vi "DriveExecute_PID_Autotune.vi"(8 "error in (no error)":errorcluster) -> (0 "error out":errorcluster)   [LabVIEW 2020]
doc: "Execute for Drie\n\nClosed control loop for drive\n\ninput: \n error in (cluster)\n\noutput:\n error out (cluster)"
uses:
  <vilib>/Rock Robotics/WPI/ThirdParty/Phoenix-LabVIEW/Motor Controller/Controls/CTRE_Phoenix_MotorControl_ControlMode.ctl
  <vilib>/Rock Robotics/WPI/ThirdParty/JAS_Junk/TrajLib/SimpleMotorFF_Calculate.vi
  <vilib>/Rock Robotics/WPI/ThirdParty/JAS_Junk/TrajLib/VI/Util_GetTime_U32.vi
  <vilib>/Rock Robotics/WPI/ThirdParty/JAS_Junk/TrajLib/PIDController_AtSetpoint.vi
  <vilib>/Rock Robotics/WPI/ThirdParty/JAS_Junk/TrajLib/PIDController_SetPIDF.vi
  <vilib>/Rock Robotics/WPI/ThirdParty/JAS_Junk/TrajLib/PIDController_SetDerivativeFilter.vi
  <vilib>/Rock Robotics/WPI/ThirdParty/JAS_Junk/TrajLib/PIDController_SetIntegratorRange.vi
  <vilib>/Rock Robotics/WPI/ThirdParty/JAS_Junk/TrajLib/PIDController_SetTolerancePandV.vi
  <vilib>/Rock Robotics/WPI/ThirdParty/JAS_Junk/TrajLib/PIDController_DisableContinousInput.vi
  <vilib>/Rock Robotics/WPI/ThirdParty/JAS_Junk/TrajLib/PIDController_EnableContinousInput.vi
  <vilib>/Rock Robotics/WPI/ThirdParty/JAS_Junk/TrajLib/PIDController_Reset.vi
  <vilib>/Rock Robotics/WPI/ThirdParty/JAS_Junk/TrajLib/PIDController_New.vi
  <vilib>/Rock Robotics/WPI/ThirdParty/JAS_Junk/TrajLib/PIDController_SetOutputLimits.vi
  <vilib>/Rock Robotics/WPI/ThirdParty/JAS_Junk/TrajLib/SlewRateLimiter_New.vi
  <vilib>/Rock Robotics/WPI/ThirdParty/JAS_Junk/TrajLib/SlewRateLimiter_Reset.vi
  <vilib>/Rock Robotics/WPI/ThirdParty/JAS_Junk/TrajLib/SlewRateLimiter_Calculate.vi
  <vilib>/Rock Robotics/WPI/ThirdParty/JAS_Junk/TrajLib/SlewRateLimiter_SetRate.vi
  <vilib>/Rock Robotics/WPI/ThirdParty/JAS_Junk/TrajLib/PIDController_NewPeriod.vi
  <vilib>/Rock Robotics/SystemInterfaces/NetworkCommunication/NetComm_UsageReport_report.vi
  <vilib>/Rock Robotics/SystemInterfaces/Utilities/FPGA_UtilitiesRead LocalTime.vi
  <vilib>/Rock Robotics/WPI/ThirdParty/JAS_Junk/TrajLib/VI/Util_GetTime_U64.vi
  DriveGlobal.vi
  <vilib>/Rock Robotics/WPI/ThirdParty/Phoenix-LabVIEW/Motor Controller/Get/CTRE_Phoenix_MotorController_GetSelectedSensorData.vi
  <vilib>/Rock Robotics/WPI/ThirdParty/JAS_Junk/TrajLib/Globals/Util_LibraryGlobals.vi
  <vilib>/Rock Robotics/WPI/ThirdParty/JAS_Junk/TrajLib/PIDController_AdvCalculate_FF_Sp_Pv.vi
  <vilib>/Rock Robotics/Network Tables/NT Write Value.vi
  <vilib>/Rock Robotics/Network Tables/NT Write Boolean.vi
  <vilib>/Rock Robotics/Network Tables/NT Write Number.vi
  <vilib>/Rock Robotics/WPI/ThirdParty/JAS_Junk/TrajLib/Trajectory_Library.lvlib
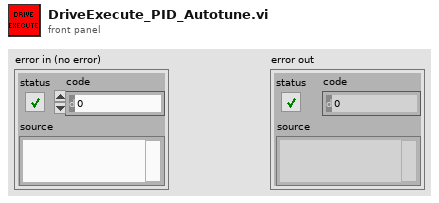
[diagram p1: front panel]
types:
  T1 = enum16{"Ziegler Nicols - Fast", "Ziegler Nicols - Normal", "Ziegler Nicols - Slow", "CHR regulator - 0% overshoot", "CHR regulator - 20% overshoot", "CHR servo - 0 % overshoot", "CHR servo - 20% overshoot"}
  T2 = typedef "CTRE_Phoenix_MotorControl_ControlMode.ctl" = u16
  T3 = typedef "WPI_MotorControlDeviceRef.ctl" = cluster{"DeviceStatus":errorcluster, "Type":T4, "PWM":cluster{"PWM Channel":T5, "DeadBand":T6}, "CAN":cluster{"Device Number":u8, "SetOutput VI Ref":variant, "GetOutput VI Ref":variant, "Enable VI Ref":variant, "Disable VI Ref":variant, "Data":variant}, "Invert":bool, "DIO PWM":cluster{"PWM \"Enable\" Channel":T5, "DIOChannel":T7, "PWM Rate":dbl}}
  T4 = typedef "WPI_MotorControlType.ctl" = enum16{"PWM", "CAN", "DIO PWM"}
  T5 = typedef "FPGA_DIOPWMChannel.ctl" = enum8{"PWM 0", "PWM 1", "PWM 2", "PWM 3", "PWM 4", "PWM 5", "PWM 6", "PWM 7", "PWM 8", "PWM 9", "PWM MXP 0", "PWM MXP 1", "PWM MXP 2", "PWM MXP 3", "PWM MXP 4", "PWM MXP 5", "PWM MXP 6", "PWM MXP 7", "PWM MXP 8", "PWM MXP 9", "Invalid"}
  T6 = typedef "WPI_PWMDeadband.ctl" = cluster{"Name":string, "maxPositivePwm":i32, "minPositivePwm":i32, "centerPwm":i32, "maxNegativePwm":i32, "minNegativePwm":i32, "angularRange":u16}
  T7 = typedef "FPGA_DIOChannel.ctl" = enum8{"DIO 0", "DIO 1", "DIO 2", "DIO 3", "DIO 4", "DIO 5", "DIO 6", "DIO 7", "DIO 8", "DIO 9", "DIO MXP 0", "DIO MXP 1", "DIO MXP 2", "DIO MXP 3", "DIO MXP 4", "DIO MXP 5", "DIO MXP 6", "DIO MXP 7", "DIO MXP 8", "DIO MXP 9", "DIO MXP 10", "DIO MXP 11", "DIO MXP 12", "DIO MXP 13", "DIO MXP 14", "DIO MXP 15", "SPI Port CS1", "SPI Port CS2", "SPI Port CS3", "SPI Port MISO", "SPI Port MOSI", "Invalid"}
  T8 = typedef "ADIS16470 Device Reference.ctl" = cluster{"DevStatus":errorcluster, "Hardware Config":T9, "Calibration Complete":refnum<notifier>, "Status Reference":refnum<data-value>, "Data Reference":refnum<data-value>, "Sychronous Process VI":T12, "Cmd FIFO":refnum<k33>, "Source":T13, "Data FIFO":refnum<k33>, "Calibration Time (ms)":u32, "Data Reference":refnum<data-value>}
  T9 = typedef "ADIS16470 Hardware Configuration.ctl" = cluster{"SPI Clock Rate (Hz)":dbl, "IMU SPI Mode (3)":T10, "IMU Reset Pin":T7, "IMU SPI Bus":T11, "IMU Data Ready Pin":T7, "Stall Config":cluster{"Pow2BytesPerRead":u8, "StallTicks":u16, "CsToSclkTicks":u8}}
  T10 = typedef "WPI_SPIMode.ctl" = enum16{"Mode 0 (Clk Idle Low,Sample on Leading)", "Mode 1 (Clk Idle Low,Sample on Trailing)", "Mode 2 (Clk Idle High,Sample on Leading)", "Mode 3 (Clk Idle High,Sample on Trailing)"}
  T11 = typedef "spi_bus.ctl" = enum16{"SPI On-Board, CS0", "SPI On-Board, CS1", "SPI On-Board, CS2", "SPI On-Board, CS3", "SPI MXP", "Invalid"}
  T12 = typedef "ADIS16470 Process.ctl" = refnum<vi>
  T13 = typedef "FPGA_CounterEncoderSourceConvertionLVSourceType.ctl" = cluster{"DevStatus":errorcluster, "AnalogTriggerMode?":bool, "DigitalMode":cluster{"DIO Channel":T14}, "AnalogTriggerMode":cluster{"AnalogTriggerIndex":T15, "OutputType":T16}}
  T14 = typedef "FPGA_DIODigitalSourceChannel.ctl" = enum8{"DIO 0", "DIO 1", "DIO 2", "DIO 3", "DIO 4", "DIO 5", "DIO 6", "DIO 7", "DIO 8", "DIO 9", "DIO MXP 0", "DIO MXP 1", "DIO MXP 2", "DIO MXP 3", "DIO MXP 4", "DIO MXP 5", "DIO MXP 6", "DIO MXP 7", "DIO MXP 8", "DIO MXP 9", "DIO MXP 10", "DIO MXP 11", "DIO MXP 12", "DIO MXP 13", "DIO MXP 14", "DIO MXP 15", "SPI Port CS1", "SPI Port CS2", "SPI Port CS3", "SPI Port MISO", "SPI Port MOSI", "Disabled"}
  T15 = typedef "FPGA_AnalogTriggerIndex.ctl" = enum8{"Trig 0", "Trig 1", "Trig 2", "Trig 3", "Trig 4", "Trig 5", "Trig 6", "Trig 7", "Invalid"}
  T16 = typedef "FPGA_AnalogTriggerOutType.ctl" = enum16{"InWindow", "TriggerState", "Rising", "Falling"}
  T17 = typedef "ADIS16470 Data.ctl" = cluster{"XAngle":dbl, "YAngle":dbl, "ZAngle":dbl}
  T18 = typedef "Trajectory_Library.lvlib/SIMPLE_MOTOR_FF.ctl" = cluster{"Ks":dbl, "Kv":dbl, "Ka":dbl, "KnInv":dbl}
  T19 = typedef "Trajectory_Library.lvlib/PID_ADV_LIMITS.ctl" = cluster{"MaxInput":dbl, "MinInput":dbl, "Continuous":bool, "MaxOutput":dbl, "MinOutput":dbl}
  T20 = typedef "Trajectory_Library.lvlib/PID_ADV_TUNING.ctl" = cluster{"Kf":dbl, "Kp":dbl, "Ki":dbl, "Kd":dbl, "MaximumIntegral":dbl, "MinimumIntegral":dbl, "Filter Derivative":bool}
  T21 = cluster{"Controller Constant Type":enum16{"Ziegler Nicols - Fast", "Ziegler Nicols - Normal", "Ziegler Nicols - Slow", "CHR regulator - 0% overshoot", "CHR regulator - 20% overshoot", "CHR servo - 0 % overshoot", "CHR servo - 20% overshoot"}, "Type of Controller":enum16{"P", "PI", "PID"}, "CO Offset":dbl, "Kn":dbl, "Tuning Tolerance":dbl, "Plant Tolerance":dbl, "Newest Avg Time ":i32, "Long Ave Time":i32}
  T22 = cluster{"Plant Gain (K)":dbl, "Time Constant (T)":dbl, "Dead Time (L)":dbl, "stimulus operating point":dbl, "response operating point":dbl}
  T23 = cluster{"proportional gain (Kp)":dbl, "integral time (Ki / Sec)":dbl, "derivative time (Kd /Sec)":dbl}
  T24 = cluster{"Const Done":bool, "Plant Done":bool, "PV Std Dev":dbl, "CO Std Dev":dbl}
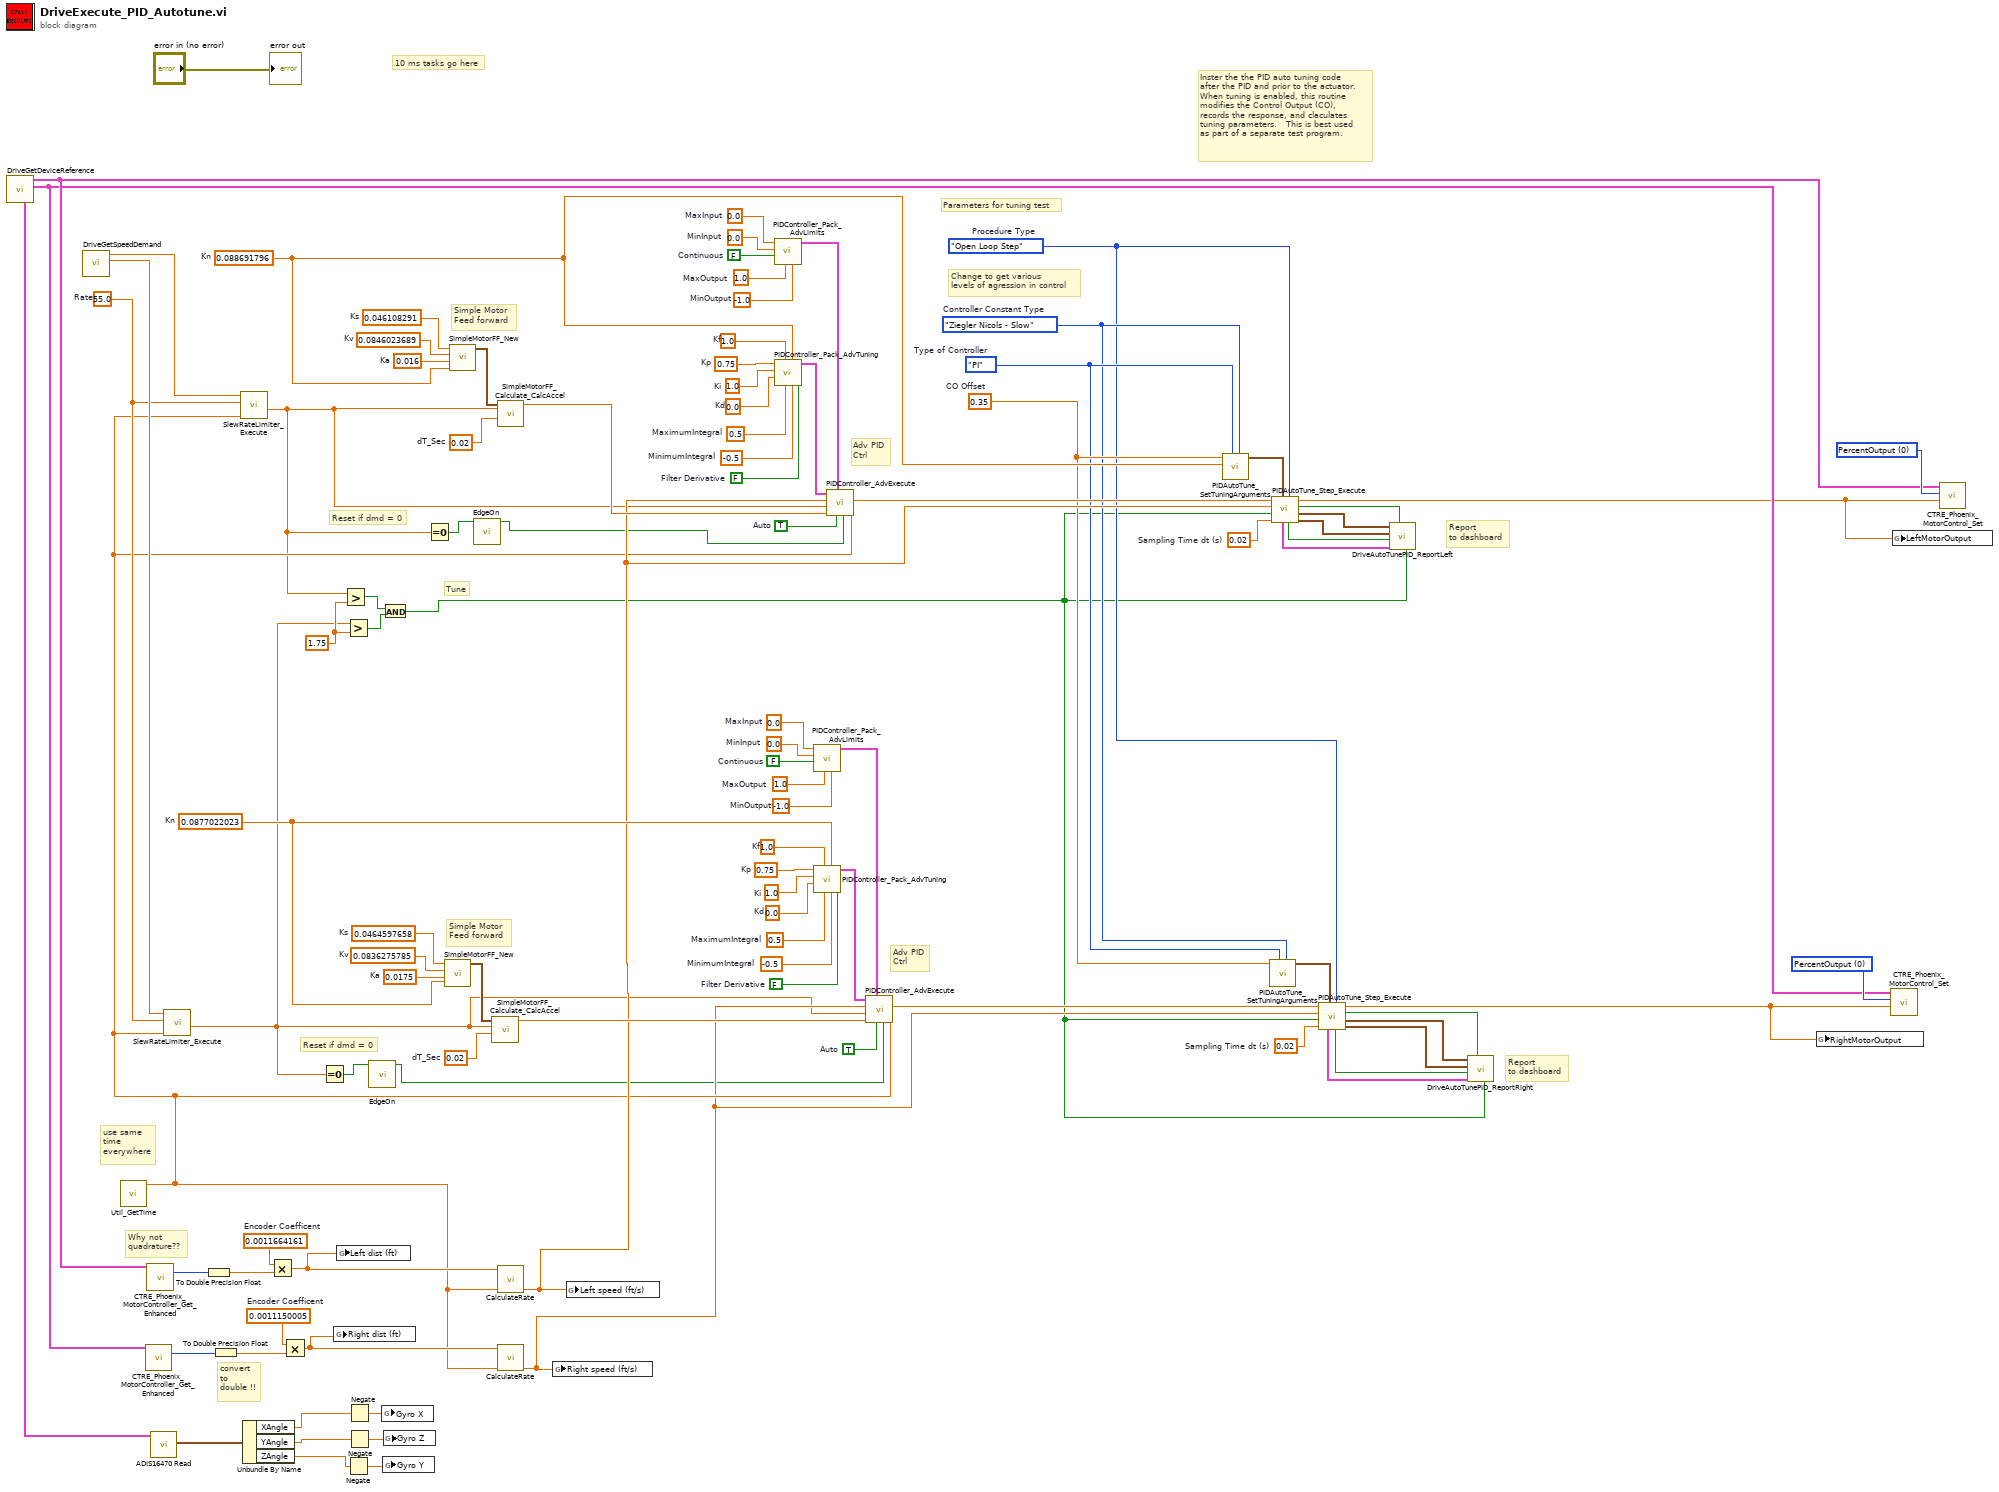
[diagram p0: block diagram]
diagram:
  w24 = enum16{"Open Loop Step", "Closed Loop Step"}."Open Loop Step"  # Procedure Type
  w25 = T1."Ziegler Nicols - Slow"  # Controller Constant Type
  w26 = enum16{"P", "PI", "PID"}."PI"  # Type of Controller
  w27 = 0.35  # CO Offset
  w21 = 1.75
  w31 = 0.02  # Sampling Time dt (s)
  w37 = 0.02  # Sampling Time dt (s)
  w42 = 55.0  # Rate
  w53 = 0.0011150005  # Encoder Coefficent
  w55 = 0.0011664161  # Encoder Coefficent
  w60 = TRUE  # Auto
  w5 = TRUE  # Auto
  w61 = 0.0877022023  # Kn
  w75 = 0.75  # Kp
  w74 = 1.0  # Ki
  w73 = 0.0  # Kd
  w72 = 1.0  # Kf
  w71 = 0.5  # MaximumIntegral
  w70 = -0.5  # MinimumIntegral
  w69 = FALSE  # Filter Derivative
  w67 = 0.0  # MinInput
  w66 = FALSE  # Continuous
  w65 = 1.0  # MaxOutput
  w68 = -1.0  # MinOutput
  w64 = 0.0  # MaxInput
  w32 = 0.088691796  # Kn
  w88 = 0.75  # Kp
  w43 = 1.0  # Ki
  w87 = 0.0  # Kd
  w86 = 1.0  # Kf
  w85 = 0.5  # MaximumIntegral
  w84 = -0.5  # MinimumIntegral
  w83 = FALSE  # Filter Derivative
  w81 = 0.0  # MinInput
  w80 = FALSE  # Continuous
  w79 = 1.0  # MaxOutput
  w82 = -1.0  # MinOutput
  w78 = 0.0  # MaxInput
  w93 = 0.02  # dT_Sec
  w91 = 0.0464597658  # Ks
  w90 = 0.0836275785  # Kv
  w89 = 0.0175  # Ka
  w98 = 0.02  # dT_Sec
  w96 = 0.046108291  # Ks
  w95 = 0.0846023689  # Kv
  w94 = 0.016  # Ka
  w102 = T2 0 items=["PercentOutput"=0, "Position"=1, "Velocity"=2, "Current"=3, "Follower"=5, "MotionProfile"=6, "MotionMagic"=7, "MotionProfileArc"=10, "Disabled"=15] ("Control Mode")
  w103 = T2 0 items=["PercentOutput"=0, "Position"=1, "Velocity"=2, "Current"=3, "Follower"=5, "MotionProfile"=6, "MotionMagic"=7, "MotionProfileArc"=10, "Disabled"=15] ("Control Mode")
  # "Reset if dmd = 0"
  # "Reset if dmd = 0"
  # "Report \nto dashboard"
  # "Report \nto dashboard"
  # "Change to get various\nlevels of agression in control"
  # "Parameters for tuning test"
  # "Tune"
  # "Inster the the PID auto tuning code\nafter the PID and prior to the actuator.\nWhen tuning is enabled, this routine\nmodifies the Control Output (CO), \nrecords the response, and claculates\ntuning parameters.   This is best used\nas part of a separate test program."
  # "convert \nto\ndouble !!"
  # "Why not\nquadrature??"
  # "use same\ntime\neverywhere"
  # "Adv PID\nCtrl"
  # "Adv PID\nCtrl"
  # "Simple Motor\nFeed forward"
  # "Simple Motor\nFeed forward"
  # "10 ms tasks go here"
  n1 = call "DriveGetDeviceReference.vi"() -> ("RightDriveTrain"=w56:T3, "LeftDriveTrain"=w57:T3, "Gryo"=w99:T8)  [unwired: 9 in]
  n2 = call "DriveGetSpeedDemand.vi"() -> ("RSpeedDemand (ft/s)"=w50:dbl, "LSpeedDemand (ft/s)"=w51:dbl)  [unwired: 10 in]
  n3 = call <vilib>:"Util_GetTime.vi"() -> ("FPGA_Time_Seconds"=w28:dbl)  [unwired: 9 in, 2 out]
  n4 = call-poly <vilib>:"CTRE_Phoenix_MotorController_Get_Enhanced.vi"("PhoenixMotorControlDevRef"=w56) -> ("Position (Raw Sensor Units)"=w41:i32)  [unwired: 11 in, 3 out]
  n5 = call-poly <vilib>:"CTRE_Phoenix_MotorController_Get_Enhanced.vi"("PhoenixMotorControlDevRef"=w57) -> ("Position (Raw Sensor Units)"=w40:i32)  [unwired: 11 in, 3 out]
  n6 = call <vilib>:"ADIS16470 Read.vi"("ADIS16470DevRef"=w99) -> ("ADIS16470 Value"=w100:T17)  [unwired: 7 in, 3 out]
  n7 = call <vilib>:"SlewRateLimiter_Execute.vi"("Time"=w28, "PositiveRate"=w42, "Input"=w50) -> ("Output"=w2:dbl)  [unwired: 7 in, 1 out]
  n8 = To Double Precision Float(number=w40) -> (double precision float=w39:dbl)
  n9 = To Double Precision Float(number=w41) -> (double precision float=w38:dbl)
  n10 = call <vilib>:"SlewRateLimiter_Execute.vi"("Time"=w28, "PositiveRate"=w42, "Input"=w51) -> ("Output"=w7:dbl)  [unwired: 7 in, 1 out]
  n11 = Unbundle By Name(w100) -> ("XAngle"=w44:dbl, "YAngle"=w46:dbl, "ZAngle"=w45:dbl)
  n12 = Multiply(x=w55, y=w39) -> (x*y=w54:dbl)
  n13 = Multiply(x=w53, y=w38) -> (x*y=w52:dbl)
  n14 = Equal To 0?(x=w2) -> (x = 0?=w3:bool)
  n15 = global write "DriveGlobal.vi" "Right dist (ft)"(w52) -> ()
  n16 = global write "DriveGlobal.vi" "Left dist (ft)"(w54) -> ()
  n17 = Greater?(x=w7, y=w21) -> (0:w20:bool)
  n18 = Greater?(x=w2, y=w21) -> (0:w19:bool)
  n19 = Negate(x=w45) -> (-x=w48:dbl)
  n20 = Negate(x=w44) -> (-x=w49:dbl)
  n21 = Negate(x=w46) -> (-x=w47:dbl)
  n22 = call "EdgeOn.vi"("Current State"=w3) -> ("Edge On Found"=w1:bool)  [unwired: 10 in]
  n23 = global write "DriveGlobal.vi" "Gyro X"(w49) -> ()
  n24 = And(x=w20, y=w19) -> (x .and. y?=w8:bool)
  n25 = global write "DriveGlobal.vi" "Gyro Y"(w48) -> ()
  n26 = global write "DriveGlobal.vi" "Gyro Z"(w47) -> ()
  n27 = Equal To 0?(x=w7) -> (x = 0?=w6:bool)
  n28 = call <vilib>:"SimpleMotorFF_New.vi"("Kn"=w61, "Ka"=w89, "Kv"=w90, "Ks"=w91) -> ("SIMPLE_MOTOR_FF"=w92:T18)  [unwired: 7 in]
  n29 = call <vilib>:"SimpleMotorFF_New.vi"("Kn"=w32, "Ka"=w94, "Kv"=w95, "Ks"=w96) -> ("SIMPLE_MOTOR_FF"=w97:T18)  [unwired: 7 in]
  n30 = call "EdgeOn.vi"("Current State"=w6) -> ("Edge On Found"=w4:bool)  [unwired: 10 in]
  n31 = call <vilib>:"SimpleMotorFF_Calculate_CalcAccel.vi"("dT_Sec"=w93, "VelSp"=w2, "SIMPLE_MOTOR_FF"=w92) -> ("FeedForward"=w58:dbl)  [unwired: 8 in]
  n32 = call <vilib>:"SimpleMotorFF_Calculate_CalcAccel.vi"("dT_Sec"=w98, "VelSp"=w7, "SIMPLE_MOTOR_FF"=w97) -> ("FeedForward"=w59:dbl)  [unwired: 8 in]
  n33 = call "CalculateRate.vi"("Time (s)"=w28, "Distance (units)"=w54) -> ("Rate (units/s)"=w34:dbl)  [unwired: 9 in]
  n34 = call "CalculateRate.vi"("Time (s)"=w28, "Distance (units)"=w52) -> ("Rate (units/s)"=w22:dbl)  [unwired: 9 in]
  n35 = global write "DriveGlobal.vi" "Right speed (ft/s)"(w22) -> ()
  n36 = global write "DriveGlobal.vi" "Left speed (ft/s)"(w34) -> ()
  n37 = call <vilib>:"PIDController_Pack_AdvLimits.vi"("MinOutput"=w82, "MaxOutput"=w79, "Continuous"=w80, "MinInput"=w81, "MaxInput"=w78) -> ("Adv PID Limits"=w76:T19)  [unwired: 6 in]
  n38 = call <vilib>:"PIDController_Pack_AdvTuning.vi"("Filter Derivative"=w83, "MinimumIntegral"=w84, "Kn"=w32, "MaximumIntegral"=w85, "Kf"=w86, "Kd"=w87, "Ki"=w43, "Kp"=w88) -> ("Adv PID Tuning"=w77:T20)  [unwired: 3 in]
  n39 = call <vilib>:"PIDController_Pack_AdvLimits.vi"("MinOutput"=w68, "MaxOutput"=w65, "Continuous"=w66, "MinInput"=w67, "MaxInput"=w64) -> ("Adv PID Limits"=w62:T19)  [unwired: 6 in]
  n40 = call <vilib>:"PIDController_Pack_AdvTuning.vi"("Filter Derivative"=w69, "MinimumIntegral"=w70, "Kn"=w61, "MaximumIntegral"=w71, "Kf"=w72, "Kd"=w73, "Ki"=w74, "Kp"=w75) -> ("Adv PID Tuning"=w63:T20)  [unwired: 3 in]
  n41 = call <vilib>:"PIDController_AdvExecute.vi"("Time"=w28, "Reset"=w4, "Auto"=w5, "Adv PID Limits"=w76, "FF-FeedForward"=w59, "SP-SetPoint"=w7, "PV-Measurement"=w34, "Adv PID Tuning"=w77) -> ("CO-ControlOutput"=w35:dbl)  [unwired: 1 in, 2 out]
  n42 = call <vilib>:"PIDController_AdvExecute.vi"("Time"=w28, "Reset"=w1, "Auto"=w60, "Adv PID Limits"=w62, "FF-FeedForward"=w58, "SP-SetPoint"=w2, "PV-Measurement"=w22, "Adv PID Tuning"=w63) -> ("CO-ControlOutput"=w29:dbl)  [unwired: 1 in, 2 out]
  n43 = call <vilib>:"PIDAutoTune_SetTuningArguments.vi"("Controller Constant Type"=w25, "Type of Controller"=w26, "Kn"=w32, "CO Offset"=w27) -> ("Configuration Parameters"=w36:T21)  [unwired: 7 in]
  n44 = call <vilib>:"PIDAutoTune_SetTuningArguments.vi"("Controller Constant Type"=w25, "Type of Controller"=w26, "CO Offset"=w27) -> ("Configuration Parameters"=w30:T21)  [unwired: 8 in]
  n45 = call <vilib>:"PIDAutoTune_Step_Execute.vi"("Procedure Type"=w24, "Configuration Parameters"=w36, "Sampling Time dt (s)"=w37, "Tune"=w8, "Measurement  (PV)"=w34, "Control Output (Co)"=w35) -> ("Plant and Test Data"=w17:T22, "New Tuning Parameters"=w18:T23, "Tuning Done"=w16:bool, "Adj CO"=w33:dbl, "Error Occured"=w15:bool, "Diagnostic Info"=w14:T24)
  n46 = call <vilib>:"PIDAutoTune_Step_Execute.vi"("Procedure Type"=w24, "Configuration Parameters"=w30, "Sampling Time dt (s)"=w31, "Tune"=w8, "Measurement  (PV)"=w22, "Control Output (Co)"=w29) -> ("Plant and Test Data"=w11:T22, "New Tuning Parameters"=w12:T23, "Tuning Done"=w13:bool, "Adj CO"=w23:dbl, "Error Occured"=w10:bool, "Diagnostic Info"=w9:T24)
  n47 = call "DriveAutoTunePID_ReportLeft.vi"("Tuning in Progress"=w8, "Tuning Done in"=w16, "Diagnostic Info in"=w14, "Error Occured in"=w15, "Plant and Test Data in"=w17, "New Tuning Parameters in"=w18) -> ()  [unwired: 6 in]
  n48 = call "DriveAutoTunePID_ReportRight.vi"("Tuning in Progress"=w8, "Tuning Done in"=w13, "Diagnostic Info in"=w9, "Error Occured in"=w10, "Plant and Test Data in"=w11, "New Tuning Parameters in"=w12) -> ()  [unwired: 6 in]
  n49 = global write "DriveGlobal.vi" "RightMotorOutput"(w23) -> ()
  n50 = call <vilib>:"CTRE_Phoenix_MotorControl_Set.vi"("Output"=w23, "Control Mode"=w102, "PhoenixMotorControlDevRef"=w56) -> ()  [unwired: 7 in, 2 out]
  n51 = global write "DriveGlobal.vi" "LeftMotorOutput"(w33) -> ()
  n52 = call <vilib>:"CTRE_Phoenix_MotorControl_Set.vi"("Output"=w33, "Control Mode"=w103, "PhoenixMotorControlDevRef"=w57) -> ()  [unwired: 7 in, 2 out]
  "error out" <- "error in (no error)"
